vi "readBFile.vi"() -> ()   [LabVIEW 2023]
panel:
  in  "?":bool
  in  "file path (use dialog)":path
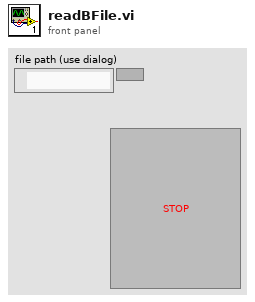
[diagram p1: front panel]
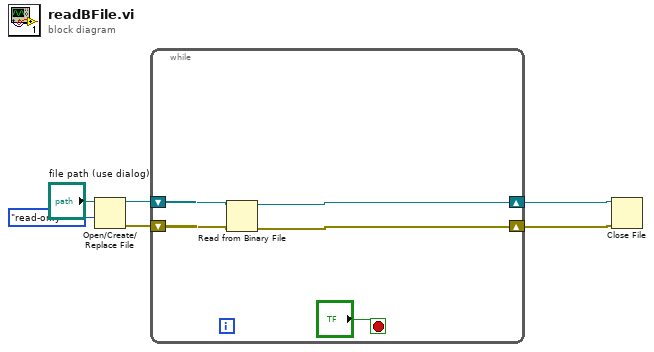
[diagram p0: block diagram]
diagram:
  n1 = Open/Create/Replace File(file path (use dialog)="file path (use dialog)", access (0:read/write)=enum16{"read/write", "read-only", "write-only"}."read-only") -> (refnum out=w5:refnum<file>, error out=w4:errorcluster)  [unwired: 4 in, 1 out]
  n2 = while {
    shift-right: [w9] -> w3
    shift-left: w5 -> [w11]
    shift-right: [w8] -> w2
    shift-left: w4 -> [w10]
    stop <- "?" stop-if-true
    n3 = Read from Binary File(8:w10, 11:w11) -> (0:w8:errorcluster, 3:w9:refnum<file>)  [unwired: 4 in, 2 out]
  }
  n4 = Close File(refnum=w3, error in=w2) -> ()  [unwired: 2 out]
